vi "sub vi - AI USB4704 (3)  Create Task v4.vi"(0 "Test":bool=TRUE, 9 "Rate Hz":dbl, 11 "Samples":dbl) -> (1 "physical channels 0":string="DemoDevice,BID#0/ai0:1" caption="property value", 2 "physical channels 1":string="DemoDevice,BID#0/ai0:1" caption="property value", 3 "physical channels 2":string="DemoDevice,BID#0/ai0:1" caption="property value", 4 "TASK USB 0":i32, 6 "TASK USB 1":i32, 8 "TASK USB 2":i32, 14 "AI Task Er":bool, 15 "error array":errorcluster[](array[cluster]))   [LabVIEW 2017]
uses:
  <userlib>/DAQNavi Polymorphic VI/create/DAQNavi Create Channel(AI-Voltage).vi
  <userlib>/DAQNavi Polymorphic VI/configure/timing/DAQNavi Timing(Convert Clock).vi
  <userlib>/DAQNavi Polymorphic VI/configure/DAQNavi Get Property/AI/DAQNaviGet_AI_ConvertClock_Rate.vi
panel:
  in  "Tab Control":enum32{"Tasks In", "USB #0", "USB #1", "USB #2"}(tab)
  out "value range 0":string="+/- 5 V" caption="property value"
  out "convert rate 0":dbl
  out "value range  1":string="+/- 5 V" caption="property value"
  out "convert rate 1":dbl
  out "value range  2":string="+/- 5 V" caption="property value"
  out "convert rate 2":dbl
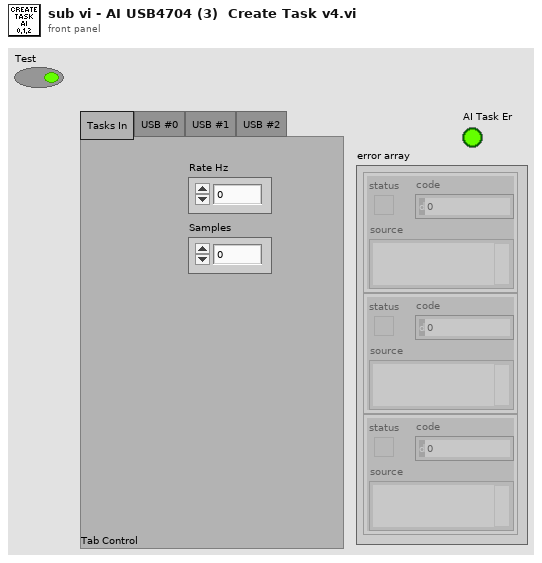
[diagram p1: front panel]
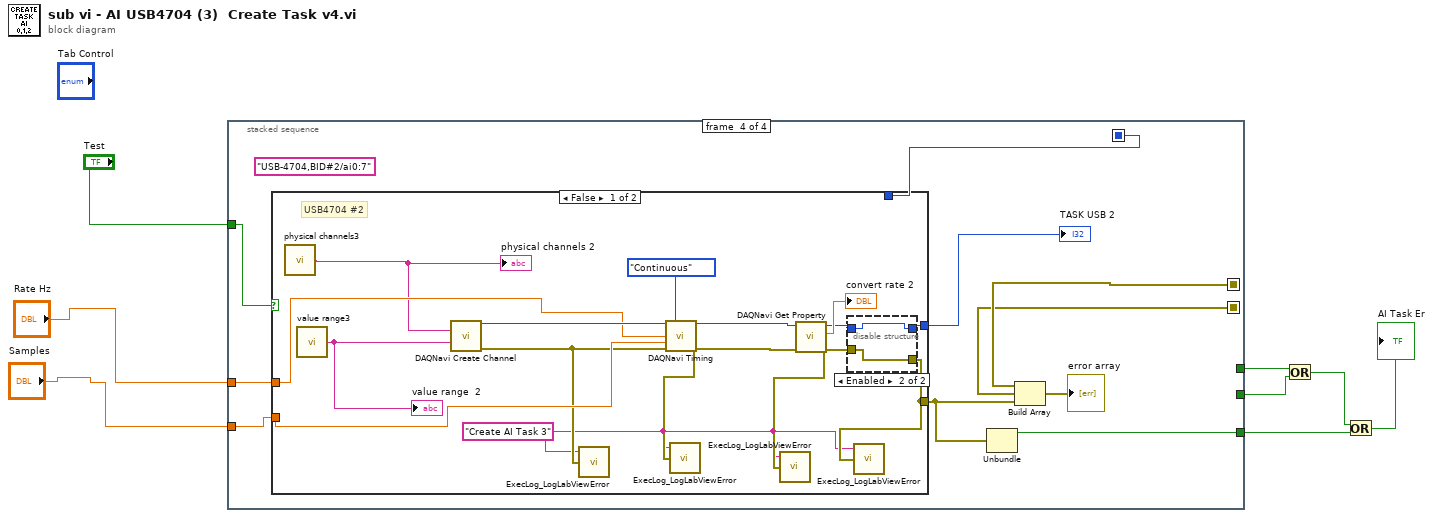
[diagram p0: block diagram]
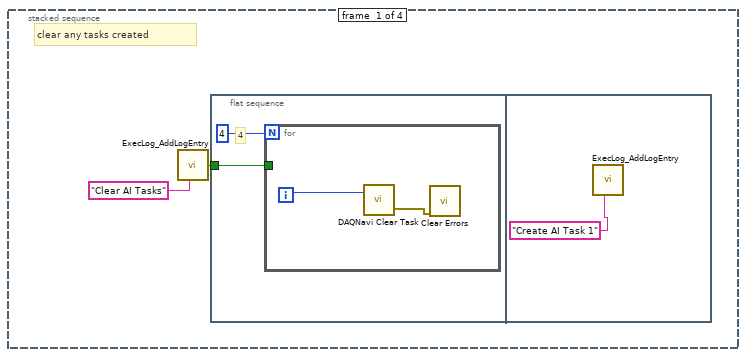
[diagram p2: hidden frame]
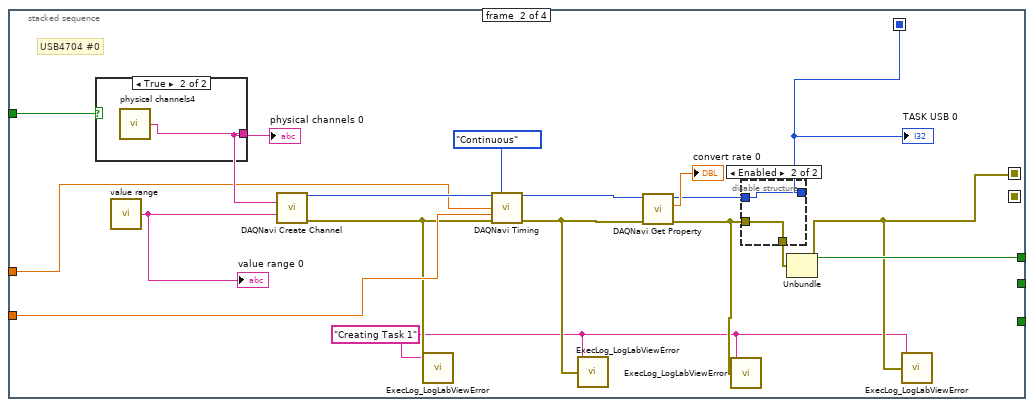
[diagram p3: hidden frame]
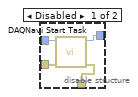
[diagram p4: hidden frame]
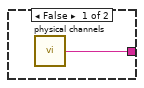
[diagram p5: hidden frame]
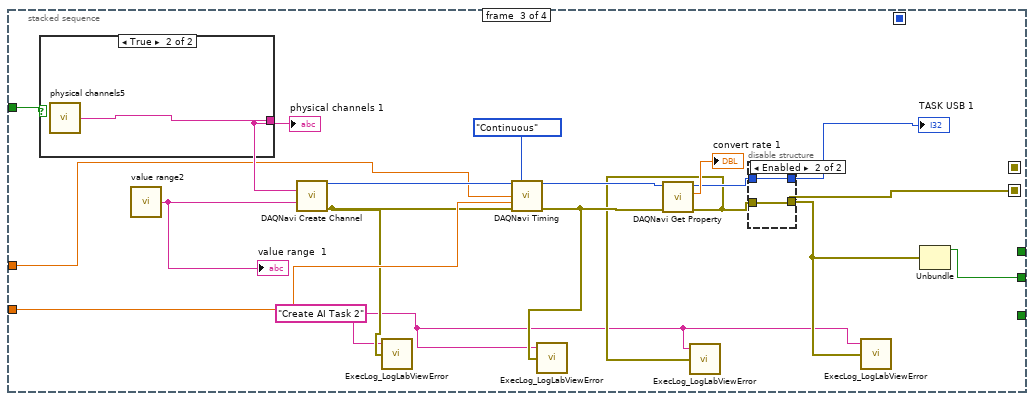
[diagram p6: hidden frame]
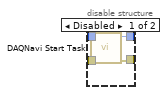
[diagram p7: hidden frame]
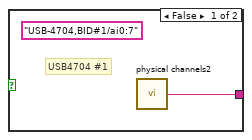
[diagram p8: hidden frame]
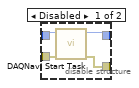
[diagram p9: hidden frame]
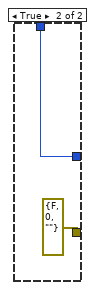
[diagram p10: hidden frame]
diagram:
  n1 = stacked-sequence {
    seq-local: [_ w17 _ _] -> [_ _ _ w75]
    seq-local: [_ _ w42 _] -> [_ _ _ w74]
    seq-local: [_ w21 _ _] -> [_ _ _ w67]
    tunnel: "Rate Hz" -> [_ w26 w51 w72]
    tunnel: "Samples" -> [_ w25 w50 w71]
    tunnel: [_ _ _ w70] -> w6
    tunnel: [_ w24 _ _] -> w5
    tunnel: [_ _ w49 _] -> w4
    tunnel: "Test" -> [_ w22 w46 w66]
    frame #0 {
      # "clear any tasks created"
      n2 = call "ExecLog_AddLogEntry.vi"("Msg"="Clear AI Tasks") -> ("NewMsg"=w9:bool)  [unwired: 7 in, 2 out]
      n3 = flat-sequence {
        tunnel: w9 -> [w11]
        frame #0 {
          # "4"
          n4 = for {
            N: 4 -> [_]
            tunnel: w11 -> [_]
            i -> [w14]
            n5 = call <userlib>:"DAQNavi Clear Task.vi"("task in"=w14) -> ("error out"=w13:errorcluster)  [unwired: 2 in]
            n6 = call <vilib>:"Clear Errors.vi"("error in (no error)"=w13) -> ()  [unwired: 5 in, 2 out]
          }
        }
        frame #1 {
          n7 = call "ExecLog_AddLogEntry.vi"("Msg"="Create AI Task 1") -> ()  [unwired: 7 in, 3 out]
        }
      }
    }
    frame #1 {
      w16 = "Creating Task 1" ("string 1")
      # "USB4704 #0"
      n8 = case shown="True" w22 {
        tunnel: [w39 w40] -> w31
        frame False {
          n9 = call "physical channels"() -> ("property value"=w39:string)  [unwired: 1 out]
        }
        frame True {
          n10 = call "physical channels4"() -> ("property value"=w40:string)  [unwired: 1 out]
        }
      }
      "physical channels 0" <- w31
      n11 = call "value range"() -> ("property value"=w32:string)  [unwired: 1 out]
      "value range 0" <- w32
      n12 = call-poly <userlib>:"DAQNavi Create Channel.vi"("physical channels"=w31, "value range"=w32) -> ("task out"=w27:i32, "error out"=w20:errorcluster)  [unwired: 3 in, 9 out]
      n13 = call "ExecLog_LogLabViewError.vi"("error IO"=w20, "string 1"=w16) -> ()  [unwired: 2 in, 1 out]
      n14 = call-poly <userlib>:"DAQNavi Timing.vi"("task in"=w27, "sample mode"=enum16{"Finite", "Continuous"}."Continuous", "rate"=w26, "samples per channel"=w25, "error in (no error)"=w20) -> ("task out"=w29:i32, "error out"=w19:errorcluster)  [unwired: 1 in, 8 out]
      n15 = call "ExecLog_LogLabViewError.vi"("error IO"=w19, "string 1"=w16) -> ()  [unwired: 2 in, 1 out]
      n16 = call-poly <userlib>:"DAQNavi Get Property.vi"("error in (no error)"=w19, "task in"=w29) -> ("error out"=w18:errorcluster, "rate"=→"convert rate 0":dbl, "task out"=w23:i32)  [unwired: 7 out]
      n17 = call "ExecLog_LogLabViewError.vi"("error IO"=w18, "string 1"=w16) -> ()  [unwired: 2 in, 1 out]
      n18 = disable-structure shown="Enabled" {
        disable-tunnel: w23 -> [w36 w38]
        disable-tunnel: [w35 w38] -> w21
        disable-tunnel: w18 -> [w34 w37]
        disable-tunnel: [w33 w37] -> w17
        frame Disabled {
          n19 = call <userlib>:"DAQNavi Start Task.vi"("error in (no error)"=w34, "task in"=w36) -> ("error out"=w33:errorcluster, "task out"=w35:i32)  [unwired: 8 in]
        }
        frame Enabled {
        }
      }
      "TASK USB 0" <- w21
      n20 = Unbundle(w17) -> ("status"=w24:bool)  [unwired: 2 out]
      n21 = call "ExecLog_LogLabViewError.vi"("error IO"=w17, "string 1"=w16) -> ()  [unwired: 2 in, 1 out]
    }
    frame #2 {
      w41 = "Create AI Task 2" ("string 1")
      n22 = case shown="True" w46 {
        tunnel: [w64 w65] -> w56
        frame False {
          (unwired) "USB-4704,BID#1/ai0:7" ("property value")
          # "USB4704 #1"
          n23 = call "physical channels2"() -> ("property value"=w64:string)  [unwired: 1 out]
        }
        frame True {
          n24 = call "physical channels5"() -> ("property value"=w65:string)  [unwired: 1 out]
        }
      }
      "physical channels 1" <- w56
      n25 = call "value range2"() -> ("property value"=w57:string)  [unwired: 1 out]
      "value range  1" <- w57
      n26 = call-poly <userlib>:"DAQNavi Create Channel.vi"("physical channels"=w56, "value range"=w57) -> ("task out"=w52:i32, "error out"=w45:errorcluster)  [unwired: 3 in, 9 out]
      n27 = call "ExecLog_LogLabViewError.vi"("error IO"=w45, "string 1"=w41) -> ()  [unwired: 2 in, 1 out]
      n28 = call-poly <userlib>:"DAQNavi Timing.vi"("task in"=w52, "sample mode"=enum16{"Finite", "Continuous"}."Continuous", "rate"=w51, "samples per channel"=w50, "error in (no error)"=w45) -> ("task out"=w54:i32, "error out"=w44:errorcluster)  [unwired: 1 in, 8 out]
      n29 = call "ExecLog_LogLabViewError.vi"("error IO"=w44, "string 1"=w41) -> ()  [unwired: 2 in, 1 out]
      n30 = call-poly <userlib>:"DAQNavi Get Property.vi"("error in (no error)"=w44, "task in"=w54) -> ("error out"=w43:errorcluster, "rate"=→"convert rate 1":dbl, "task out"=w48:i32)  [unwired: 7 out]
      n31 = call "ExecLog_LogLabViewError.vi"("error IO"=w43, "string 1"=w41) -> ()  [unwired: 2 in, 1 out]
      n32 = disable-structure shown="Enabled" {
        disable-tunnel: w48 -> [w61 w63]
        disable-tunnel: [w60 w63] -> w47
        disable-tunnel: w43 -> [w59 w62]
        disable-tunnel: [w58 w62] -> w42
        frame Disabled {
          n33 = call <userlib>:"DAQNavi Start Task.vi"("error in (no error)"=w59, "task in"=w61) -> ("error out"=w58:errorcluster, "task out"=w60:i32)  [unwired: 8 in]
        }
        frame Enabled {
        }
      }
      "TASK USB 1" <- w47
      n34 = call "ExecLog_LogLabViewError.vi"("error IO"=w42, "string 1"=w41) -> ()  [unwired: 2 in, 1 out]
      n35 = Unbundle(w42) -> ("status"=w49:bool)  [unwired: 2 out]
    }
    frame #3 {
      (unwired) "USB-4704,BID#2/ai0:7" ("property value")
      n36 = case shown="False" w66 {
        tunnel: w72 -> [w85 _]
        tunnel: w71 -> [w84 _]
        tunnel: [w82 w97] -> w69
        tunnel: [w77 errorcluster {"status"=FALSE, "code"=0, "source"=""} ("error out")] -> w68
        tunnel: w67 -> [_ w97]
        frame False {
          w76 = "Create AI Task 3" ("string 1")
          # "USB4704 #2"
          n37 = call "physical channels3"() -> ("property value"=w81:string)  [unwired: 1 out]
          "physical channels 2" <- w81
          n38 = call "value range3"() -> ("property value"=w90:string)  [unwired: 1 out]
          "value range  2" <- w90
          n39 = call-poly <userlib>:"DAQNavi Create Channel.vi"("physical channels"=w81, "value range"=w90) -> ("task out"=w86:i32, "error out"=w80:errorcluster)  [unwired: 3 in, 9 out]
          n40 = call "ExecLog_LogLabViewError.vi"("error IO"=w80, "string 1"=w76) -> ()  [unwired: 2 in, 1 out]
          n41 = call-poly <userlib>:"DAQNavi Timing.vi"("task in"=w86, "sample mode"=enum16{"Finite", "Continuous"}."Continuous", "rate"=w85, "samples per channel"=w84, "error in (no error)"=w80) -> ("task out"=w88:i32, "error out"=w79:errorcluster)  [unwired: 1 in, 8 out]
          n42 = call "ExecLog_LogLabViewError.vi"("error IO"=w79, "string 1"=w76) -> ()  [unwired: 2 in, 1 out]
          n43 = call-poly <userlib>:"DAQNavi Get Property.vi"("error in (no error)"=w79, "task in"=w88) -> ("error out"=w78:errorcluster, "rate"=→"convert rate 2":dbl, "task out"=w83:i32)  [unwired: 7 out]
          n44 = call "ExecLog_LogLabViewError.vi"("error IO"=w78, "string 1"=w76) -> ()  [unwired: 2 in, 1 out]
          n45 = disable-structure shown="Enabled" {
            disable-tunnel: w83 -> [w94 w96]
            disable-tunnel: [w93 w96] -> w82
            disable-tunnel: w78 -> [w92 w95]
            disable-tunnel: [w91 w95] -> w77
            frame Disabled {
              n46 = call <userlib>:"DAQNavi Start Task.vi"("error in (no error)"=w92, "task in"=w94) -> ("error out"=w91:errorcluster, "task out"=w93:i32)  [unwired: 8 in]
            }
            frame Enabled {
            }
          }
          n47 = call "ExecLog_LogLabViewError.vi"("error IO"=w77, "string 1"=w76) -> ()  [unwired: 2 in, 1 out]
        }
        frame True {
        }
      }
      "TASK USB 2" <- w69
      n48 = Unbundle(w68) -> ("status"=w70:bool)  [unwired: 2 out]
      n49 = Build Array(w75, w74, w68) -> (→"error array":errorcluster[])
    }
  }
  n50 = Or(x=w5, y=w4) -> (x .or. y?=w7:bool)
  n51 = Or(x=w7, y=w6) -> (x .or. y?=→"AI Task Er":bool)
